vi "excelReport2.vi"(6 "device":string, 7 "customer":string, 8 "Shift":string(combo), 9 "End Date":string="2014/9/24", 11 "From Date":string="2014/9/20") -> ()   [LabVIEW 2012]
uses:
  <vilib>/Utility/NIReport.llb/Generate Report Object Reference.ctl
  <vilib>/Utility/NIReport.llb/NI_report.lvclass
  <vilib>/addons/database/Auxilliary.llb/DB Tools Cursor Type.ctl
  <vilib>/addons/database/Connection.llb/DB Tools Open Connec (Path).vi
  <vilib>/addons/database/Connection.llb/Conn Execute.vi
  <vilib>/addons/database/Recordset.llb/Rec Fetch Recordset Data (R).vi
  <vilib>/addons/database/Recordset.llb/Rec Destroy - Connection.vi
  <vilib>/Utility/NIReport.llb/Append Text Table to Report (wrap).vi
  <vilib>/addons/database/_DB Variant To Data/Database Variant To Data.xnode
  <vilib>/addons/database/NI_Database_API.lvlib
  <vilib>/Utility/NIReport.llb/Excel/NI_Excel.lvclass
  <vilib>/addons/_office/NI_ReportGenerationToolkit.lvlib
panel:
  in  "Running":string[][](table)
  in  "Report Template":path=path "c:/m100/data/AT.xls"
  out "report out":T1
  out "error out":errorcluster
  out "Row Headers":string[](array[string])
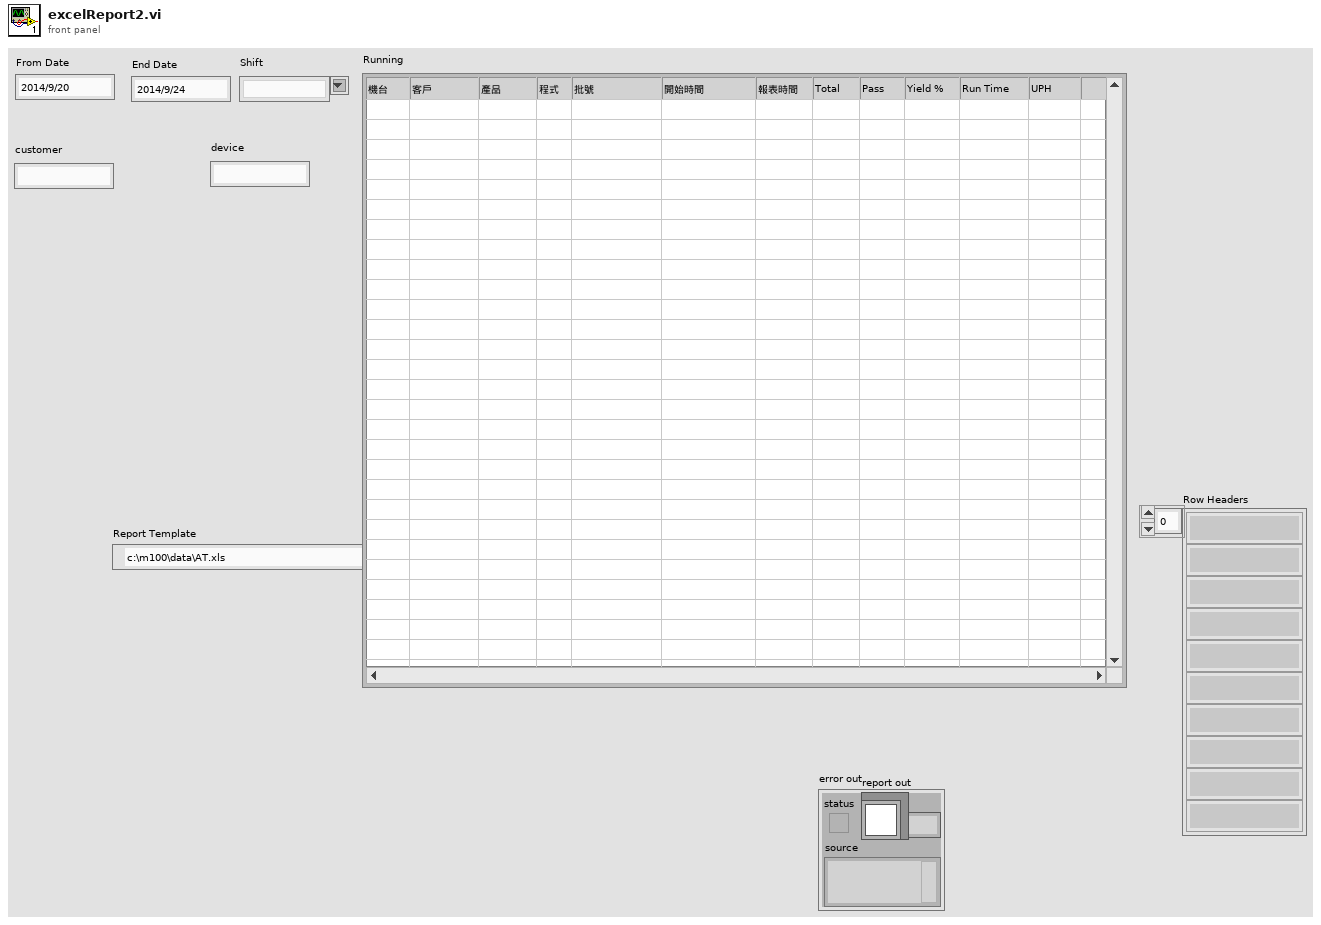
[diagram p1: front panel]
types:
  T1 = typedef "Generate Report Object Reference.ctl" = refnum<class "NI_report.lvclass">
  T2 = typedef "NI_Database_API.lvlib/DB Tools Cursor Type.ctl" = enum16{"forward-only", "keyset", "dynamic", "static"}
  T3 = typedef "NI_Database_API.lvlib/Conn ObjectReference.ctl" = refnum<k1>
  T4 = typedef "NI_Database_API.lvlib/Rec ObjectReference.ctl" = refnum<k1>
  T5 = enum16{"Standard Report", "HTML", "Word", "Excel"}
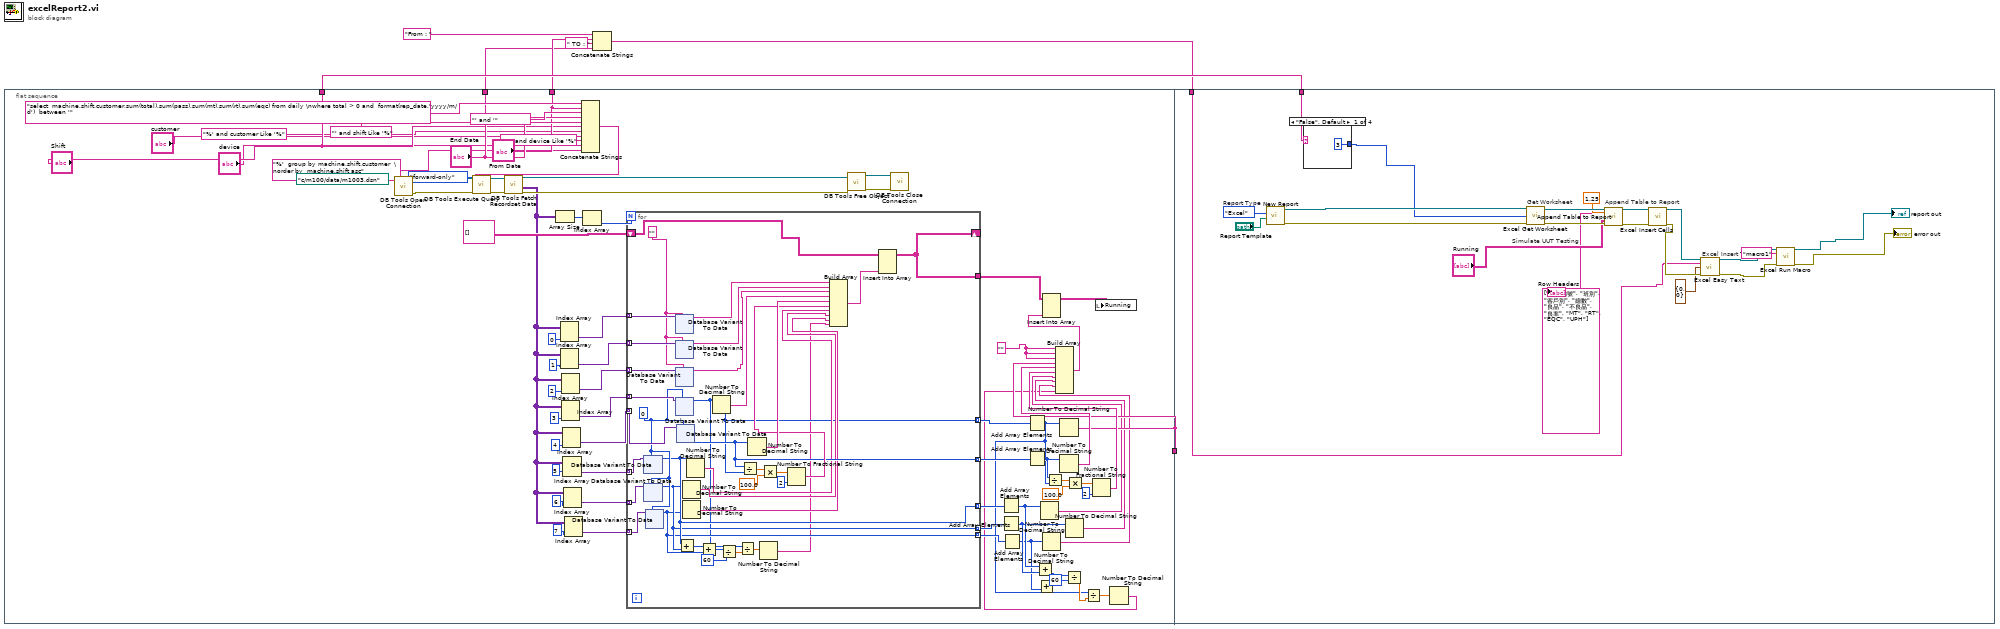
[diagram p0: block diagram]
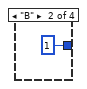
[diagram p2: hidden frame]
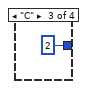
[diagram p3: hidden frame]
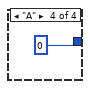
[diagram p4: hidden frame]
diagram:
  n1 = flat-sequence {
    tunnel: [w43] -> w7
    tunnel: ["Shift"] -> w6
    tunnel: ["From Date"] -> w4
    tunnel: ["End Date"] -> w2
    tunnel: w7 -> [_]
    tunnel: w6 -> [w379]
    tunnel: w1 -> [w377]
    frame #0 {
      w60 = "" ("element")
      n2 = call-poly <vilib>:"DB Tools Open Connection.vi"("connection information"=path "c:/m100/data/m1003.dsn") -> ("error out"=w48:errorcluster, "connection reference"=w49:T3)  [unwired: 7 in]
      n3 = Concatenate Strings("select  machine,shift,customer,sum(total),sum(pass),sum(mt),sum(rt),sum(eqc) from daily \nwhere total > 0 and  format(rep_date,'yyyy/m/d')  between '" ("string"), "From Date", "' and '" ("string"), "End Date", "' and shift Like '%" ("string"), "Shift", "%' and customer Like '%" ("string"), "customer", "%' and device Like '%" ("string"), "device", "%'  group by machine,shift,customer  \norder by  machine,shift asc" ("string")) -> (w45:string)
      n4 = call-poly <vilib>:"DB Tools Execute Query.vi"("error in (no error)"=w48, "cursor type"=DB_Tools_Cursor_Type."forward-only", "SQL query"=w45, "connection reference"=w49) -> ("error out"=w51:errorcluster, "recordset reference"=w50:T4)  [unwired: 4 in]
      n5 = call-poly <vilib>:"DB Tools Fetch Recordset Data.vi"("error in (no error)"=w51, "recordset reference"=w50) -> ("error out"=w47:errorcluster, "recordset data"=w32:variant[][], "recordset reference out"=w46:T4)  [unwired: 3 in]
      n6 = Array Size(array=w32) -> (size(s)=w77:i32[])
      n7 = Index Array(array=w32, index (col)=0) -> (element=w70:variant[])  [unwired: 1 in]
      n8 = Index Array(array=w32, index (col)=1) -> (element=w69:variant[])  [unwired: 1 in]
      n9 = Index Array(array=w32, index (col)=2) -> (element=w65:variant[])  [unwired: 1 in]
      n10 = Index Array(array=w32, index (col)=3) -> (element=w68:variant[])  [unwired: 1 in]
      n11 = Index Array(array=w32, index (col)=4) -> (element=w67:variant[])  [unwired: 1 in]
      n12 = Index Array(array=w32, index (col)=5) -> (element=w31:variant[])  [unwired: 1 in]
      n13 = Index Array(array=w32, index (col)=6) -> (element=w30:variant[])  [unwired: 1 in]
      n14 = Index Array(array=w32, index (col)=7) -> (element=w29:variant[])  [unwired: 1 in]
      n15 = Index Array(array=w77) -> (element=w76:i32)  [unwired: 1 in]
      n16 = for {
        N: w76 -> [_]
        tunnel: w67 -> [w115] mode=indexing
        shift-right: [w96] -> _
        shift-left: string[][] [] -> [w100]
        tunnel: w70 -> [w114] mode=indexing
        tunnel: w69 -> [w113] mode=indexing
        tunnel: w68 -> [w112] mode=indexing
        tunnel: w65 -> [w109] mode=indexing
        tunnel: [w81] -> w19 mode=indexing
        tunnel: [w102] -> w63 mode=indexing
        tunnel: [w96] -> w41
        tunnel: w31 -> [w95] mode=indexing
        tunnel: w30 -> [w94] mode=indexing
        tunnel: w29 -> [w93] mode=indexing
        tunnel: [w85] -> w26 mode=indexing
        tunnel: [w87] -> w27 mode=indexing
        tunnel: [w88] -> w28 mode=indexing
        w92 = 0
        w108 = ""
        n17 = xnode "Database Variant To Data"("database variant"=w95, "type"=w92) -> ("data"=w88:i32)  [unwired: 1 in, 1 out]
        n18 = xnode "Database Variant To Data"("database variant"=w94, "type"=w92) -> ("data"=w87:i32)  [unwired: 1 in, 1 out]
        n19 = xnode "Database Variant To Data"("database variant"=w93, "type"=w92) -> ("data"=w85:i32)  [unwired: 1 in, 1 out]
        n20 = xnode "Database Variant To Data"("database variant"=w114, "type"=w108) -> ("data"=w99:string)  [unwired: 1 in, 1 out]
        n21 = xnode "Database Variant To Data"("database variant"=w113, "type"=w108) -> ("data"=w98:string)  [unwired: 1 in, 1 out]
        n22 = xnode "Database Variant To Data"("database variant"=w112, "type"=w92) -> ("data"=w81:i32)  [unwired: 1 in, 1 out]
        n23 = xnode "Database Variant To Data"("database variant"=w109, "type"=w108) -> ("data"=w97:string)  [unwired: 1 in, 1 out]
        n24 = xnode "Database Variant To Data"("database variant"=w115, "type"=w92) -> ("data"=w102:i32)  [unwired: 1 in, 1 out]
        n25 = Add(x=w88, y=w87) -> (x+y=w86:i32)
        n26 = Number To Decimal String(number=w87) -> (decimal integer string=w90:string)  [unwired: 1 in]
        n27 = Number To Decimal String(number=w85) -> (decimal integer string=w89:string)  [unwired: 1 in]
        n28 = Number To Decimal String(number=w88) -> (decimal integer string=w91:string)  [unwired: 1 in]
        n29 = Add(x=w86, y=w85) -> (x+y=w84:i32)
        n30 = Number To Decimal String(number=w81) -> (decimal integer string=w106:string)  [unwired: 1 in]
        n31 = Divide(x=w84, y=60) -> (x/y=w82:dbl)
        n32 = Divide(x=w81, y=w82) -> (x/y=w80:dbl)
        n33 = Divide(x=w102, y=w81) -> (x/y=w110:dbl)
        n34 = Number To Decimal String(number=w102) -> (decimal integer string=w107:string)  [unwired: 1 in]
        n35 = Number To Decimal String(number=w80) -> (decimal integer string=w79:string)  [unwired: 1 in]
        n36 = Multiply(x=w110, y=100.0) -> (x*y=w105:dbl)
        n37 = Number To Fractional String(number=w105, precision (6)=i16 2) -> (F-format string=w104:string)  [unwired: 2 in]
        n38 = Build Array(w99, w98, w97, w106, w107, w104, w91, w90, w89, w79) -> (w101:string[])
        n39 = Insert Into Array(array=w100, new element=w101) -> (w96:string[][])  [unwired: 2 in]
      }
      n40 = call-poly <vilib>:"DB Tools Free Object.vi"("error in (no error)"=w47, "recordset reference"=w46) -> ("error out"=w52:errorcluster, "connection reference"=w53:T3)  [unwired: 8 in]
      n41 = call <vilib>:"DB Tools Close Connection.vi"("error in (no error)"=w52, "connection reference"=w53) -> ()  [unwired: 5 in, 1 out]
      n42 = Add Array Elements(numeric array=w28) -> (sum=w22:i32)
      n43 = Add Array Elements(numeric array=w27) -> (sum=w21:i32)
      n44 = Add Array Elements(numeric array=w26) -> (sum=w20:i32)
      n45 = Add Array Elements(numeric array=w19) -> (sum=w13:i32)
      n46 = Add Array Elements(numeric array=w63) -> (sum=w55:i32)
      n47 = Add(x=w22, y=w21) -> (x+y=w18:i32)
      n48 = Add(x=w18, y=w20) -> ()  [unwired: 1 out]
      n49 = Number To Decimal String(number=w22) -> (decimal integer string=w25:string)  [unwired: 1 in]
      n50 = Number To Decimal String(number=w20) -> (decimal integer string=w23:string)  [unwired: 1 in]
      n51 = Divide(x=w55, y=w13) -> (x/y=w58:dbl)
      n52 = Number To Decimal String(number=w13) -> (decimal integer string=w43:string)  [unwired: 1 in]
      n53 = Number To Decimal String(number=w55) -> (decimal integer string=w62:string)  [unwired: 1 in]
      n54 = Number To Decimal String(number=w21) -> (decimal integer string=w24:string)  [unwired: 1 in]
      n55 = Divide(x=w18, y=60) -> (x/y=w16:dbl)
      n56 = Multiply(x=w58, y=100.0) -> (x*y=w57:dbl)
      n57 = Divide(x=w13, y=w16) -> (x/y=w15:dbl)
      n58 = Number To Fractional String(number=w57, precision (6)=i16 2) -> (F-format string=w54:string)  [unwired: 2 in]
      n59 = Number To Decimal String(number=w15) -> (decimal integer string=w14:string)  [unwired: 1 in]
      n60 = Build Array(w60, w60, w60, w43, w62, w54, w25, w24, w23, w14) -> (w61:string[])
      n61 = Insert Into Array(array=w41, new element=w61) -> (w42:string[][])  [unwired: 2 in]
      n62 = local write "Running"(w42) -> ()
    }
    frame #1 {
      w387 = string[] ["機台編號", "班別", "客戶別", "總數", "良品", "不良品", "良率", "MT", "RT", "EQC", "UPH"] ("row headers")
      w393 = T5."Excel"  # Report Type
      # "Excel Insert Text"
      # "Simulate UUT Testing"
      # "Append Table to Report"
      # "Get Worksheet"
      n63 = call <vilib>:"New Report.vi"("report type"=w393, "template (empty)"="Report Template") -> ("report out"=w381:refnum<class "NI_report.lvclass">, "error out"=w380:errorcluster)  [unwired: 12 in]
      n64 = case shown="\"False\", Default" w379 {
        tunnel: [3 1 2 0] -> w378
        frame "False", Default {
        }
        frame "B" {
        }
        frame "C" {
        }
        frame "A" {
        }
      }
      n65 = call <vilib>:"Excel Get Worksheet.vi"("report in"=w381, "worksheet index (0)"=w378, "error in (no error)"=w380) -> ("report out"=w391:refnum<class "NI_report.lvclass">, "error out"=w390:errorcluster)  [unwired: 11 in]
      n66 = call-poly <vilib>:"Append Table to Report.vi"("report in"=w391, "column width (1)"=1.25, "column headers"=w387, "text data"="Running", "error in (no error)"=w390) -> ("report out"=w386:refnum<class "NI_report.lvclass">, "error out"=w385:errorcluster)  [unwired: 7 in, 2 out]
      n67 = call <vilib>:"Excel Insert Cells.vi"("report in"=w386, "error in (no error)"=w385) -> ("report out"=w384:refnum<class "NI_report.lvclass">, "error out"=w383:errorcluster)  [unwired: 12 in]
      n68 = call <vilib>:"Excel Easy Text.vi"("report in"=w384, "text"=w377, "start (-1, -1)"=cluster{"row":i32, "column":i32} {"row"=0, "column"=0} ("end (-1, -1)"), "error in (no error)"=w383) -> ("report out"=w376:refnum<class "NI_report.lvclass">, "error out"=w374:errorcluster)  [unwired: 7 in, 3 out]
      n69 = call <vilib>:"Excel Run Macro.vi"("report in"=w376, "macro name"="macro1", "error in (no error)"=w374) -> ("report out"=→"report out":refnum<class "NI_report.lvclass">, "error out"=→"error out":errorcluster)  [unwired: 10 in, 1 out]
      "Row Headers" <- w387
    }
  }
  n70 = Concatenate Strings("From : " ("string"), w4, " TO : " ("string"), w2) -> (w1:string)
